vi "Teleop.vi"(10 "Match Info":T1={"Autonomous Elapsed Seconds"=0.0, "TeleOp Elapsed Seconds"=0.0, "Disabled Elapsed Seconds"=0.0, "Visited Autonomous"=FALSE, "Visited TeleOp"=FALSE, "Visited Disabled"=FALSE, "Autonomous Settings"={"Autonomous Style"=enum."Independent", "VI Refnum"=refnum}}, 11 "Call Context":T2) -> ()   [LabVIEW 2019]
doc: "This VI is called for each enabled TeleOp packet received from the DS. It is typically used to read from joysticks and other inputs and update I/O or setpoints for timed control loops. It should complete and return within 20 milliseconds or risk missing DS packets."
uses:
  <vilib>/Rock Robotics/WPI/DriverStation/WPI_DriverStationDerivedRobotMode.ctl
  <vilib>/Rock Robotics/WPI/DriverStation/WPI_DriverStationMatch Info.ctl
  Framework/Robot Global Data.vi
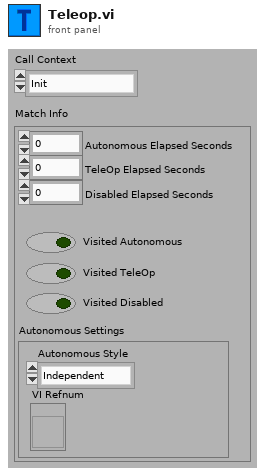
[diagram p1: front panel]
types:
  T1 = typedef "WPI_DriverStationMatch Info.ctl" = cluster{"Autonomous Elapsed Seconds":dbl, "TeleOp Elapsed Seconds":dbl, "Disabled Elapsed Seconds":dbl, "Visited Autonomous":bool, "Visited TeleOp":bool, "Visited Disabled":bool, "Autonomous Settings":cluster{"Autonomous Style":enum16{"Iterative", "Independent"}, "VI Refnum":refnum<vi>}}
  T2 = typedef "WPI_DriverStationDerivedRobotMode.ctl" = enum16{"Init", "Execute", "Stop"}
  T3 = typedef "Command Status Info.ctl" = cluster{"Name":string, "Status":T4, "notifier out":T5}
  T4 = typedef "Completion Status.ctl" = enum16{"Successful", "Aborted", "Incomplete"}
  T5 = typedef "Completion Notifier.ctl" = refnum<notifier>
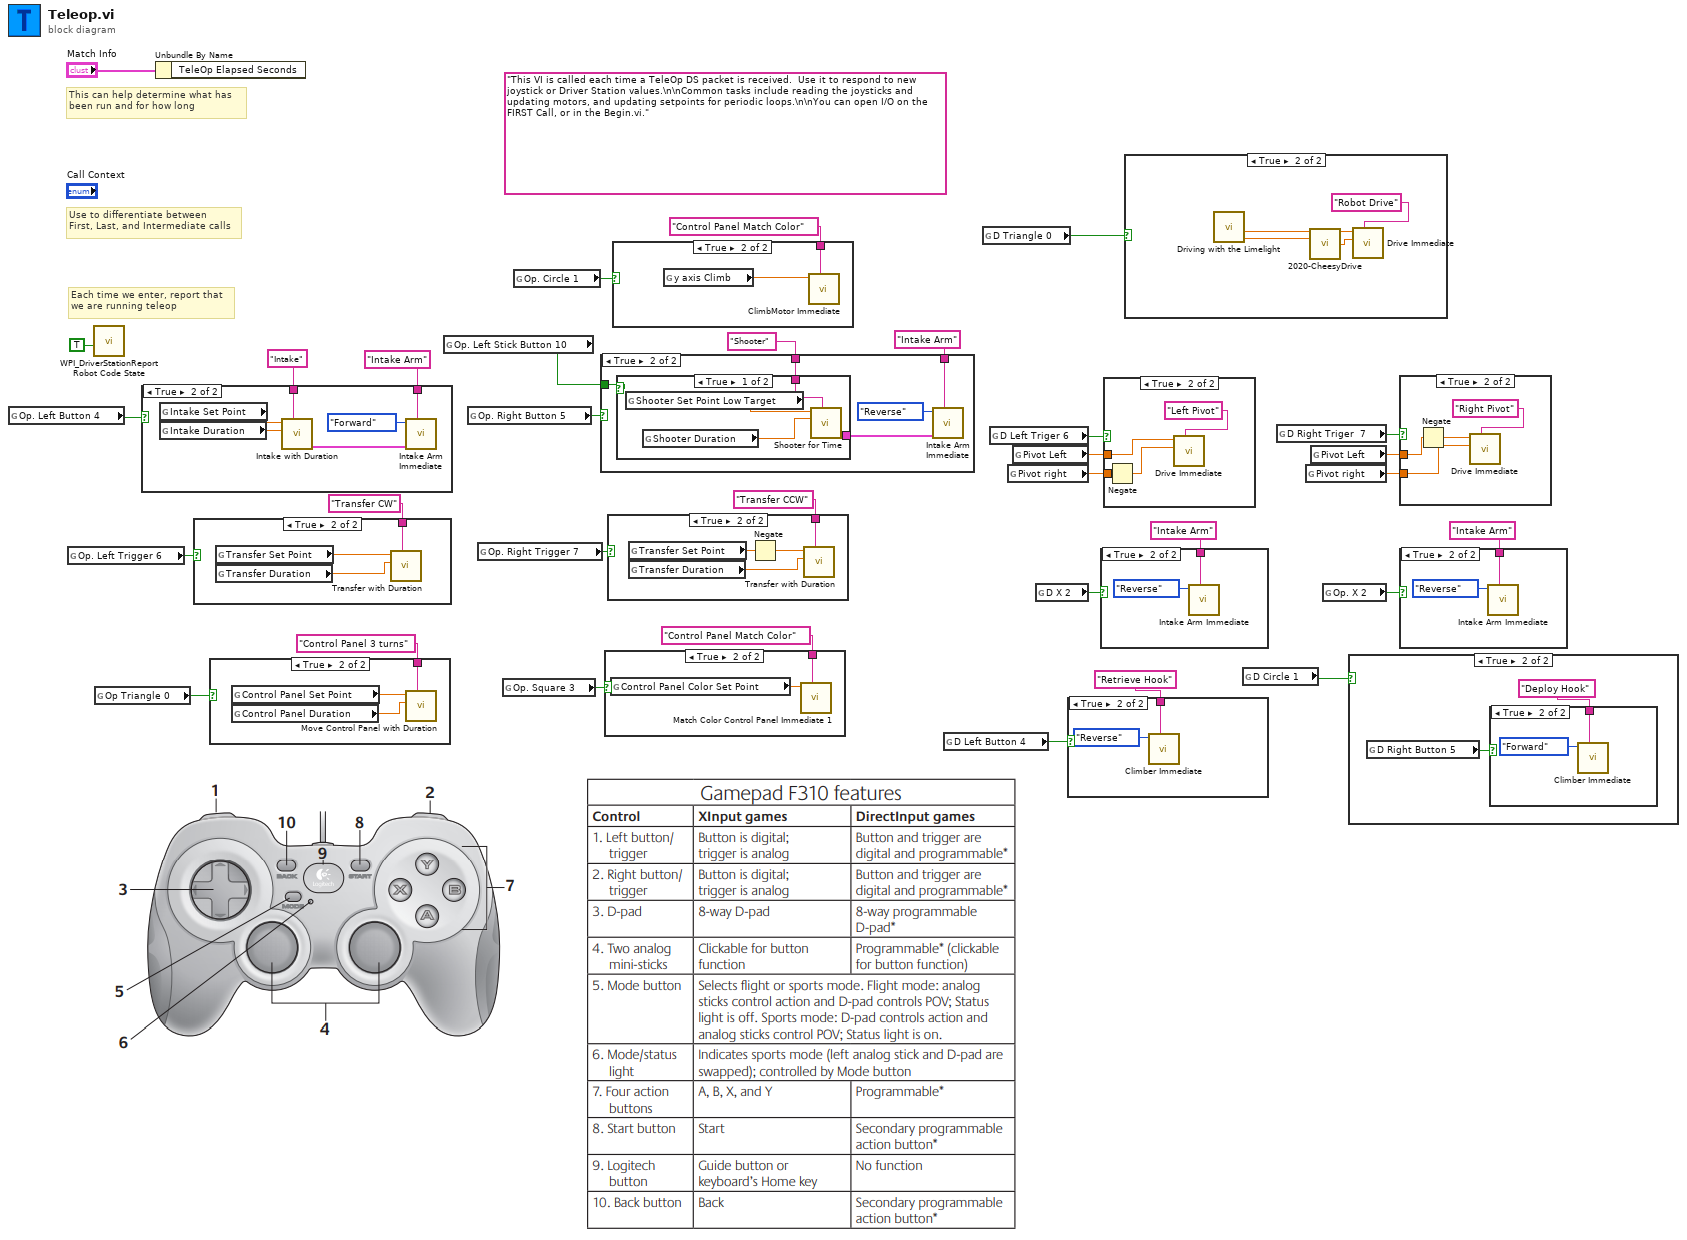
[diagram p0: block diagram]
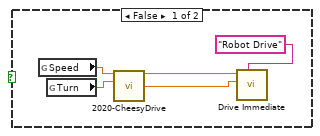
[diagram p7: hidden frame]
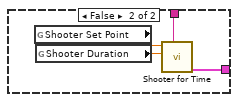
[diagram p16: hidden frame]
diagram:
  (unwired) "This VI is called each time a TeleOp DS packet is received.  Use it to respond to new joystick or Driver Station values.\n\nCommon tasks include reading the joysticks and updating motors, and updating setpoints for periodic loops.\n\nYou can open I/O on the FIRST Call, or in the Begin.vi."
  # "Each time we enter, report that\nwe are running teleop"
  # "Use to differentiate between\nFirst, Last, and Intermediate calls"
  # "This can help determine what has\nbeen run and for how long"
  n1 = global read "Robot Global Data.vi" "Op. Left Button 4"() -> (w31:bool)
  n2 = global read "Robot Global Data.vi" "Op. Left Trigger 6"() -> (w25:bool)
  n3 = call <vilib>:"WPI_DriverStationReport Robot Code State.vi"("TeleOp"=TRUE ("Autonomous")) -> ()  [unwired: 10 in, 1 out]
  n4 = global read "Robot Global Data.vi" "Op Triangle 0"() -> (w18:bool)
  n5 = case shown="True" w31 {
    tunnel: "Intake" ("refnum name") -> [_ w39]
    tunnel: "Intake Arm" ("refnum name") -> [_ w35]
    frame False {
    }
    frame True {
      n6 = global read "Robot Global Data.vi" "Intake Set Point"() -> (w38:dbl)
      n7 = global read "Robot Global Data.vi" "Intake Duration"() -> (w37:dbl)
      n8 = call "Intake with Duration.vi"("Description"=w39, "Duration (s)"=w37, "Setpoint"=w38) -> ("Command Info Out"=w34:T3)  [unwired: 8 in]
      n9 = call "Intake Arm Immediate.vi"("Description"=w35, "Command Info In"=w34, "Relay Value"=enum16{"Off", "On", "Forward", "Reverse"}."Forward") -> ()  [unwired: 8 in, 1 out]
    }
  }
  n10 = Unbundle By Name("Match Info") -> ()  [unwired: 1 out]
  n11 = case shown="True" w25 {
    tunnel: "Transfer CW" ("refnum name") -> [_ w42]
    frame False {
    }
    frame True {
      n12 = global read "Robot Global Data.vi" "Transfer Set Point"() -> (w41:dbl)
      n13 = global read "Robot Global Data.vi" "Transfer Duration"() -> (w40:dbl)
      n14 = call "Transfer with Duration.vi"("Description"=w42, "Duration (s)"=w40, "Setpoint"=w41) -> ()  [unwired: 8 in, 1 out]
    }
  }
  n15 = case shown="True" w18 {
    tunnel: "Control Panel 3 turns" ("refnum name") -> [_ w45]
    frame False {
    }
    frame True {
      n16 = global read "Robot Global Data.vi" "Control Panel Set Point"() -> (w44:dbl)
      n17 = global read "Robot Global Data.vi" "Control Panel Duration"() -> (w43:dbl)
      n18 = call "Move Control Panel with Duration.vi"("Description"=w45, "Duration (s)"=w43, "Setpoint"=w44) -> ()  [unwired: 8 in, 1 out]
    }
  }
  n19 = global read "Robot Global Data.vi" "Op. Left Stick Button 10"() -> (w1:bool)
  n20 = global read "Robot Global Data.vi" "Op. Right Button 5"() -> (w27:bool)
  n21 = global read "Robot Global Data.vi" "Op. Right Trigger 7"() -> (w26:bool)
  n22 = global read "Robot Global Data.vi" "Op. Square 3"() -> (w15:bool)
  n23 = global read "Robot Global Data.vi" "Op. Circle 1"() -> (w3:bool)
  n24 = case shown="True" w27 {
    tunnel: "Shooter" ("refnum name") -> [_ w50]
    tunnel: "Intake Arm" ("refnum name") -> [_ w48]
    tunnel: w1 -> [_ w46]
    frame False {
    }
    frame True {
      n25 = case shown="True" w46 {
        tunnel: w50 -> [w54 w58]
        tunnel: [w51 w55] -> w47
        frame True {
          n26 = global read "Robot Global Data.vi" "Shooter Set Point Low Target"() -> (w53:dbl)
          n27 = global read "Robot Global Data.vi" "Shooter Duration"() -> (w52:dbl)
          n28 = call "Shooter for Time.vi"("Description"=w54, "Duration (s)"=w52, "Setpoint"=w53) -> ("Command Info Out"=w51:T3)  [unwired: 8 in]
        }
        frame False {
          n29 = global read "Robot Global Data.vi" "Shooter Set Point"() -> (w57:dbl)
          n30 = global read "Robot Global Data.vi" "Shooter Duration"() -> (w56:dbl)
          n31 = call "Shooter for Time.vi"("Description"=w58, "Duration (s)"=w56, "Setpoint"=w57) -> ("Command Info Out"=w55:T3)  [unwired: 8 in]
        }
      }
      n32 = call "Intake Arm Immediate.vi"("Description"=w48, "Command Info In"=w47, "Relay Value"=enum16{"Off", "On", "Forward", "Reverse"}."Reverse") -> ()  [unwired: 8 in, 1 out]
    }
  }
  n33 = case shown="True" w15 {
    tunnel: "Control Panel Match Color" ("refnum name") -> [_ w60]
    frame False {
    }
    frame True {
      n34 = global read "Robot Global Data.vi" "Control Panel Color Set Point"() -> (w59:dbl)
      n35 = call "Match Color Control Panel Immediate 1.vi"("Description"=w60, "Setpoint"=w59) -> ()  [unwired: 9 in, 1 out]
    }
  }
  n36 = case shown="True" w26 {
    tunnel: "Transfer CCW" ("refnum name") -> [_ w64]
    frame False {
    }
    frame True {
      n37 = global read "Robot Global Data.vi" "Transfer Set Point"() -> (w62:dbl)
      n38 = global read "Robot Global Data.vi" "Transfer Duration"() -> (w61:dbl)
      n39 = Negate(x=w62) -> (-x=w63:dbl)
      n40 = call "Transfer with Duration.vi"("Description"=w64, "Duration (s)"=w61, "Setpoint"=w63) -> ()  [unwired: 8 in, 1 out]
    }
  }
  n41 = case shown="True" w3 {
    tunnel: "Control Panel Match Color" ("refnum name") -> [_ w66]
    frame False {
    }
    frame True {
      n42 = global read "Robot Global Data.vi" "y axis Climb"() -> (w65:dbl)
      n43 = call "ClimbMotor Immediate.vi"("Description"=w66, "Setpoint"=w65) -> ()  [unwired: 9 in, 1 out]
    }
  }
  n44 = global read "Robot Global Data.vi" "D Left Button 4"() -> (w8:bool)
  n45 = global read "Robot Global Data.vi" "D Triangle 0"() -> (w9:bool)
  n46 = global read "Robot Global Data.vi" "D Left Triger 6"() -> (w23:bool)
  n47 = global read "Robot Global Data.vi" "Pivot right"() -> (w12:dbl)
  n48 = global read "Robot Global Data.vi" "Pivot Left"() -> (w13:dbl)
  n49 = global read "Robot Global Data.vi" "D X 2"() -> (w16:bool)
  n50 = case shown="True" w8 {
    tunnel: "Retrieve Hook" ("refnum name") -> [_ w67]
    frame False {
    }
    frame True {
      n51 = call "Climber Immediate.vi"("Description"=w67, "Value"=enum16{"Off", "On", "Forward", "Reverse"}."Reverse" ("Relay Value")) -> ()  [unwired: 9 in, 1 out]
    }
  }
  n52 = case shown="True" w16 {
    tunnel: "Intake Arm" ("refnum name") -> [_ w69]
    frame False {
    }
    frame True {
      n53 = call "Intake Arm Immediate.vi"("Description"=w69, "Relay Value"=enum16{"Off", "On", "Forward", "Reverse"}."Reverse") -> ()  [unwired: 9 in, 1 out]
    }
  }
  n54 = case shown="True" w23 {
    tunnel: w13 -> [_ w73]
    tunnel: w12 -> [_ w72]
    frame False {
    }
    frame True {
      n55 = Negate(x=w72) -> (-x=w71:dbl)
      n56 = call "Drive Immediate.vi"("Description"="Left Pivot", "Right Setpoint"=w71, "Left Setpoint"=w73) -> ()  [unwired: 8 in, 1 out]
    }
  }
  n57 = case shown="True" w9 {
    frame False {
      n58 = global read "Robot Global Data.vi" "Speed"() -> (w76:dbl)
      n59 = global read "Robot Global Data.vi" "Turn"() -> (w77:dbl)
      n60 = call "2020-CheesyDrive.vi"("Throttle"=w76, "Wheel"=w77) -> ("Left PWM"=w78:dbl, "Right PWM"=w79:dbl)  [unwired: 12 in]
      n61 = call "Drive Immediate.vi"("Description"="Robot Drive", "Right Setpoint"=w79, "Left Setpoint"=w78) -> ()  [unwired: 8 in, 1 out]
    }
    frame True {
      n62 = call "Driving with the Limelight.vi"() -> ("TurnCommand"=w80:dbl, "SpeedCommand"=w81:dbl)  [unwired: 9 in, 1 out]
      n63 = call "2020-CheesyDrive.vi"("Throttle"=w81, "Wheel"=w80) -> ("Left PWM"=w83:dbl, "Right PWM"=w84:dbl)  [unwired: 12 in]
      n64 = call "Drive Immediate.vi"("Description"="Robot Drive", "Right Setpoint"=w84, "Left Setpoint"=w83) -> ()  [unwired: 8 in, 1 out]
    }
  }
  n65 = global read "Robot Global Data.vi" "D Circle 1"() -> (w2:bool)
  n66 = global read "Robot Global Data.vi" "D Right Triger  7"() -> (w22:bool)
  n67 = global read "Robot Global Data.vi" "Pivot right"() -> (w10:dbl)
  n68 = global read "Robot Global Data.vi" "Pivot Left"() -> (w11:dbl)
  n69 = global read "Robot Global Data.vi" "Op. X 2"() -> (w6:bool)
  n70 = case shown="True" w2 {
    frame False {
    }
    frame True {
      n71 = global read "Robot Global Data.vi" "D Right Button 5"() -> (w85:bool)
      n72 = case shown="True" w85 {
        tunnel: "Deploy Hook" ("refnum name") -> [_ w87]
        frame False {
        }
        frame True {
          n73 = call "Climber Immediate.vi"("Description"=w87, "Value"=enum16{"Off", "On", "Forward", "Reverse"}."Forward" ("Relay Value")) -> ()  [unwired: 9 in, 1 out]
        }
      }
    }
  }
  n74 = case shown="True" w22 {
    tunnel: w11 -> [_ w91]
    tunnel: w10 -> [_ w90]
    frame False {
    }
    frame True {
      n75 = Negate(x=w91) -> (-x=w89:dbl)
      n76 = call "Drive Immediate.vi"("Description"="Right Pivot", "Right Setpoint"=w90, "Left Setpoint"=w89) -> ()  [unwired: 8 in, 1 out]
    }
  }
  n77 = case shown="True" w6 {
    tunnel: "Intake Arm" ("refnum name") -> [_ w93]
    frame False {
    }
    frame True {
      n78 = call "Intake Arm Immediate.vi"("Description"=w93, "Relay Value"=enum16{"Off", "On", "Forward", "Reverse"}."Reverse") -> ()  [unwired: 9 in, 1 out]
    }
  }
